vi "New CHM Wizard.vi"(9 "Title":string, 11 "Base CHM Directory":path) -> ()   [LabVIEW 2015]
uses:
  Wizard/Wizard State.ctl
  <vilib>/Utility/config.llb/Write Key (String).vi
  <vilib>/Utility/config.llb/Write Key (Path).vi
  <vilib>/Utility/config.llb/NI_LVConfig.lvlib
panel:
  in  "Tab Control":T1(tab)
  in  "Default Topic Name":string
  in  "Previous":bool
  in  "Cancel":bool
  in  "Next":bool
  # "Welcome to the Compiled Help Menu Wizard."
  # "This will add the CHM Generator to your project and create a new auto-populating folder\nfor your Compiled Help Menu source files."
  # "Choose a title for your Compiled Help Menu"
  # "Choose an empty directory for your Compiled  HTML Help source files."
  # "Choose a name for the default topic of your Compiled HTML Help file. \nThis will be generated in the directory you specified."
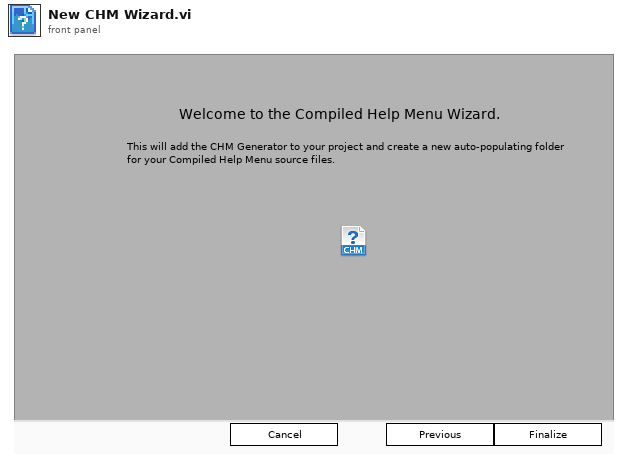
[diagram p1: front panel]
types:
  T1 = enum32{"Welcome", "Choose CHM Title", "Choose Base Path", "Choose Default Topic Name"}
  T2 = typedef "Wizard State.ctl" = enum16{"Initialize", "Wait for User", "Finalize"}
  T3 = enum8{"Enabled", "Disabled", "Disabled and Grayed Out"}
  T4 = typedef "NI_LVConfig.lvlib/Config Data RefNum.ctl" = refnum<k1>
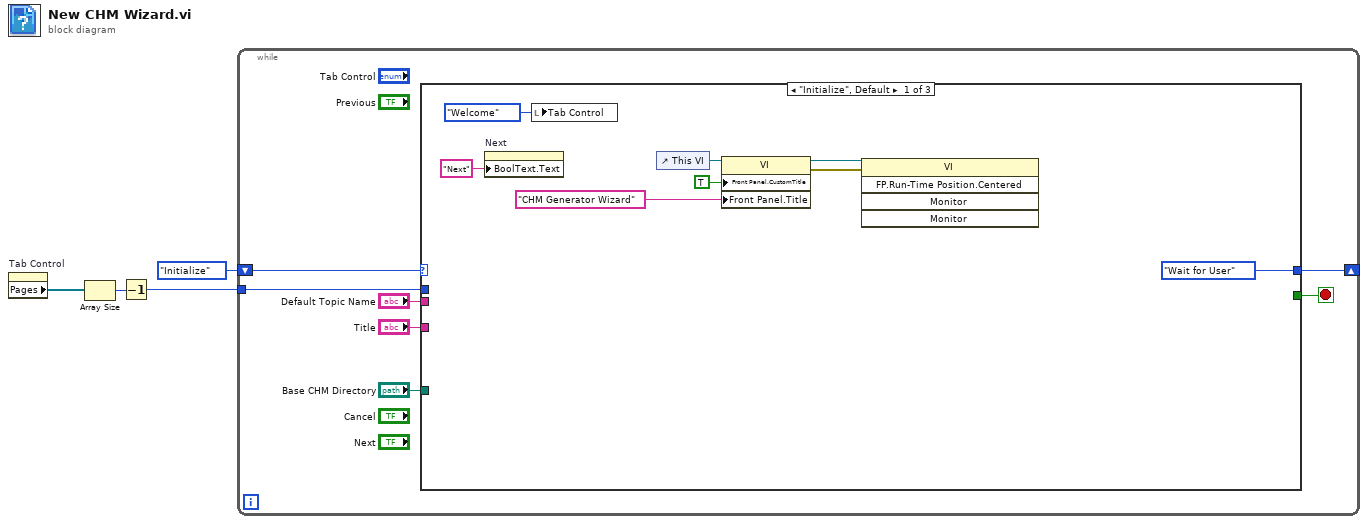
[diagram p0: block diagram]
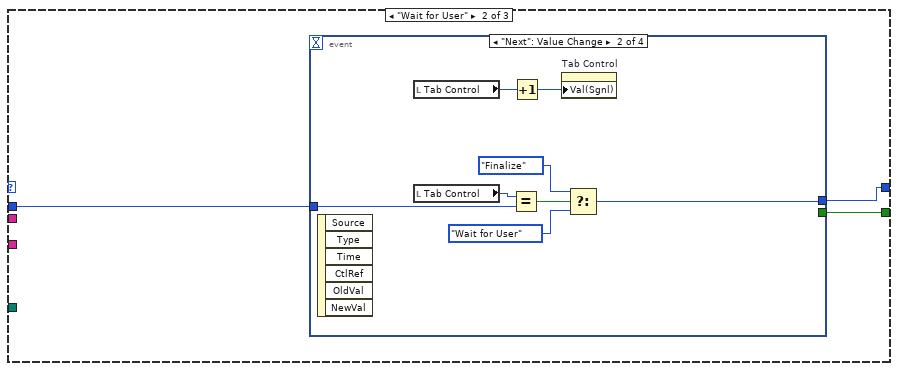
[diagram p2: hidden frame]
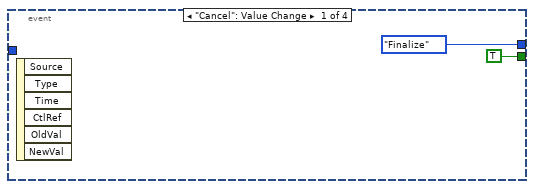
[diagram p3: hidden frame]
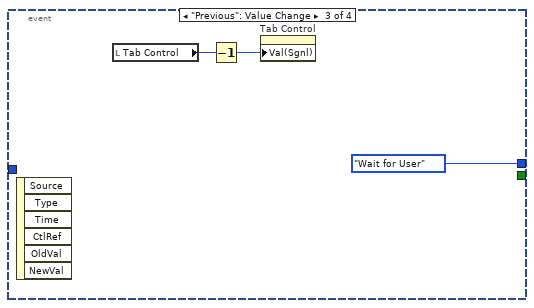
[diagram p4: hidden frame]
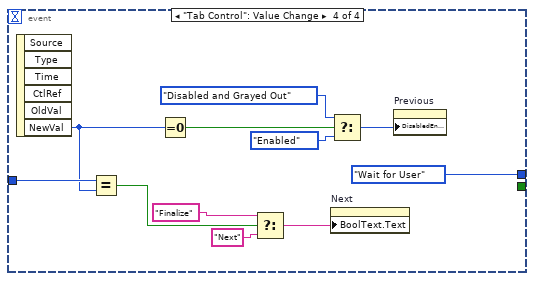
[diagram p5: hidden frame]
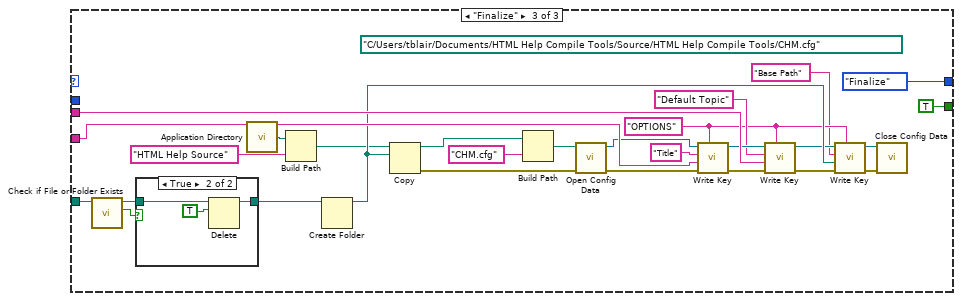
[diagram p6: hidden frame]
diagram:
  n1 = property on="Tab Control" class="TabCtl (strict)"() -> ("Pages"=w3:refnum<vi>[])  [unwired: 2 in, 2 out]
  n2 = Array Size(array=w3) -> (size(s)=w2:i32)
  n3 = Decrement(x=w2) -> (x-1=w1:i32)
  n4 = while {
    shift-right: [w10] -> _
    shift-left: Wizard_State."Initialize" -> [w11]
    tunnel: w1 -> [w8]
    stop <- w9 stop-if-true
    n5 = case shown="\"Initialize\", Default" w11 {
      tunnel: [Wizard_State."Wait for User" w21 Wizard_State."Finalize"] -> w10
      tunnel: [_ w22 TRUE] -> w9
      tunnel: w8 -> [_ w20 _]
      tunnel: "Base CHM Directory" -> [_ _ w70]
      tunnel: "Title" -> [_ _ w72]
      tunnel: "Default Topic Name" -> [_ _ w71]
      frame "Initialize", Default {
        n6 = property on="Next" class="Bool"("BoolText.Text"="Next" ("Boolean Text.Text")) -> ()  [unwired: 2 in, 2 out]
        n7 = local write "Tab Control"(T1."Welcome" ("Tab Control")) -> ()
        n8 = control-ref of="This VI"() -> (w17:refnum<vi>)
        n9 = property class="VI"(reference=w17, "Front Panel.CustomTitle"=TRUE ("Front Panel Window:Custom Title"), "Front Panel.Title"="CHM Generator Wizard" ("Front Panel Window:Title")) -> (reference out=w13:refnum<vi>, error out=w12:errorcluster)  [unwired: 1 in]
        n10 = invoke class="VI" method="FP.Run-Time Position.Centered"(reference=w13, error in=w12) -> ()  [unwired: 3 in, 5 out]
      }
      frame "Wait for User" {
        n11 = event shown="[1] \"Next\": Value Change" {
          selector: _ -> [_ _ _ _]
          dyn-events: _ -> [_ _ _ _]
          timeout: _ -> [_ _ _ _]
          tunnel: [TRUE _ _ _] -> w22
          tunnel: [Wizard_State."Finalize" w25 Wizard_State."Wait for User" Wizard_State."Wait for User"] -> w21
          tunnel: w20 -> [_ w29 _ w42]
          event "Cancel": Value Change {
            n12 = event-data() -> ()  [unwired: 1 in, 6 out]
          }
          event "Next": Value Change {
            n13 = event-data() -> ()  [unwired: 1 in, 6 out]
            n14 = local read "Tab Control"() -> (w32:T1)
            n15 = local read "Tab Control"() -> (w30:T1)
            n16 = Equal?(x=w30, y=w29) -> (x = y?=w26:bool)
            n17 = Increment(x=w32) -> (x+1=w31:T1)
            n18 = property on="Tab Control" class="TabCtl (strict)"("Val(Sgnl)"=w31) -> ()  [unwired: 2 in, 2 out]
            n19 = Select(t=Wizard_State."Finalize", s=w26, f=Wizard_State."Wait for User") -> (s? t:f=w25:T2)
          }
          event "Previous": Value Change {
            n20 = event-data() -> ()  [unwired: 1 in, 6 out]
            n21 = local read "Tab Control"() -> (w35:T1)
            n22 = Decrement(x=w35) -> (x-1=w34:T1)
            n23 = property on="Tab Control" class="TabCtl (strict)"("Val(Sgnl)"=w34) -> ()  [unwired: 2 in, 2 out]
          }
          event "Tab Control": Value Change {
            n24 = event-data() -> ("NewVal"=w41:T1)  [unwired: 1 in, 5 out]
            n25 = Equal?(x=w42, y=w41) -> (x = y?=w40:bool)
            n26 = Equal To 0?(x=w41) -> (x = 0?=w46:bool)
            n27 = Select(t="Finalize", s=w40, f="Next" ("Boolean Text.Text")) -> (s? t:f=w37:string)
            n28 = property on="Next" class="Bool"("BoolText.Text"=w37) -> ()  [unwired: 2 in, 2 out]
            n29 = Select(t=T3."Disabled and Grayed Out", s=w46, f=T3."Enabled" ("Disabled")) -> (s? t:f=w43:T3)
            n30 = property on="Previous" class="Bool"("DisabledEnum"=w43) -> ()  [unwired: 2 in, 2 out]
          }
        }
      }
      frame "Finalize" {
        w58 = "OPTIONS" ("section")
        (unwired) path "C:/Users/tblair/Documents/HTML Help Compile Tools/Source/HTML Help Compile Tools/CHM.cfg" ("Path")
        n31 = call <vilib>:"Check if File or Folder Exists.vi"("path"=w70) -> ("file or folder exists?"=w68:bool, "dup path"=w69:path)  [unwired: 8 in, 1 out]
        n32 = case shown="True" w68 {
          tunnel: w69 -> [w75 w77]
          tunnel: [w75 w76] -> w67
          frame False {
          }
          frame True {
            n33 = Delete(path (use dialog)=w77, entire hierarchy (F)=TRUE) -> (deleted path=w76:path)  [unwired: 3 in, 2 out]
          }
        }
        n34 = call <vilib>:"Application Directory.vi"() -> ("Application Directory"=w52:path)
        n35 = Build Path(base path=w52, name or relative path="HTML Help Source") -> (appended path=w50:path)
        n36 = Create Folder(path (use dialog)=w67) -> (created path=w66:path)  [unwired: 2 in, 2 out]
        n37 = Copy(10:w66, 11:w50) -> (0:w59:errorcluster, 3:w49:path)  [unwired: 3 in, 1 out]
        n38 = Build Path(base path=w49, name or relative path="CHM.cfg") -> (appended path=w47:path)
        n39 = call <vilib>:"Open Config Data.vi"("error in (no error)"=w59, "configuration file path"=w47) -> ("error out"=w65:errorcluster, "refnum"=w64:T4)  [unwired: 7 in, 1 out]
        n40 = call-poly <vilib>:"Write Key.vi"("section"=w58, "error in (no error)"=w65, "value"=w72, "key"="Title", "refnum"=w64) -> ("error out"=w62:errorcluster, "refnum out"=w61:T4)  [unwired: 4 in, 1 out]
        n41 = call-poly <vilib>:"Write Key.vi"("section"=w58, "error in (no error)"=w62, "value"=w71, "key"="Default Topic", "refnum"=w61) -> ("error out"=w57:errorcluster, "refnum out"=w55:T4)  [unwired: 4 in, 1 out]
        n42 = call-poly <vilib>:"Write Key.vi"("section"=w58, "error in (no error)"=w57, "value"=w66, "key"="Base Path", "refnum"=w55) -> ("error out"=w56:errorcluster, "refnum out"=w54:T4)  [unwired: 4 in, 1 out]
        n43 = call <vilib>:"Close Config Data.vi"("error in (no error)"=w56, "refnum"=w54) -> ()  [unwired: 8 in, 2 out]
      }
    }
  }
